vi "GetDiscoveryInfo.vi"(7 "LabVIEW Web Service Request":refnum<class "Web Request.lvclass">) -> ()   [LabVIEW 2017]
uses:
  <vilib>/wsapi/Web Request.lvclass
  <vilib>/addons/InsightCM/Devices/Shared/Ble/BleComm/BleComm.lvlib
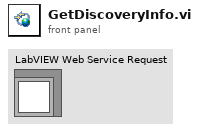
[diagram p1: front panel]
types:
  T1 = typedef "Bluetooth Sensing.lvlib/Endpoints.ctl" = cluster{"BleAddress":string, "Type":string, "Timestamp":dbl, "Properties":cluster{"Key":string, "Value":string}[]}
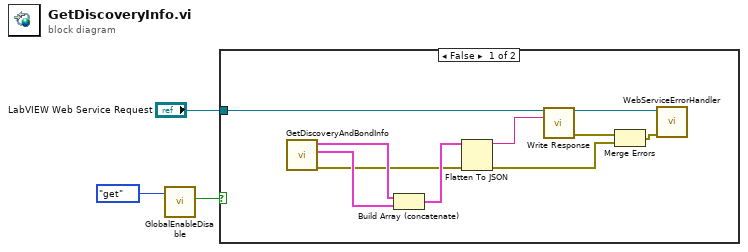
[diagram p0: block diagram]
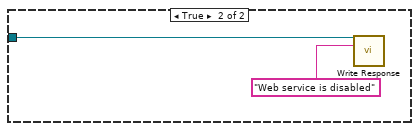
[diagram p2: hidden frame]
diagram:
  n1 = call "GlobalEnableDisable.vi"("action"=enum16{"init", "set", "get"}."get") -> ("DisableDeviceWebService"=w1:bool)  [unwired: 10 in]
  n2 = case shown="False" w1 {
    tunnel: "LabVIEW Web Service Request" -> [w13 w14]
    frame False {
      n3 = call <vilib>:"GetDiscoveryAndBondInfo.vi"() -> ("error out"=w4:errorcluster, "bonded endpoints"=w6:T1[], "discovered endpoints"=w7:T1[])  [unwired: 9 in]
      n4 = Build Array (concatenate)(w7, w6) -> (w5:T1[])
      n5 = Flatten To JSON(anything=w5, error in (no error)=w4) -> (JSON string=w9:string, 11:w8:errorcluster)  [unwired: 1 in]
      n6 = call <vilib>:"Write Response.vi"("LabVIEW Web Service Request"=w13, "response string"=w9) -> ("LabVIEW Web Service Request out"=w12:refnum<class "Web Request.lvclass">, "error out"=w11:errorcluster)  [unwired: 12 in]
      n7 = Merge Errors(w11, w8) -> (w10:errorcluster)
      n8 = call "WebServiceErrorHandler.vi"("LabVIEW Web Service Request"=w12, "error in (no error)"=w10) -> ()  [unwired: 12 in, 2 out]
    }
    frame True {
      n9 = call <vilib>:"Write Response.vi"("LabVIEW Web Service Request"=w14, "response string"="Web service is disabled") -> ()  [unwired: 12 in, 2 out]
    }
  }
